vi "GetSetParameterValues.vi"(0 "VISA resource name":refnum<visa-resource-name>, 1 "get/set":T4, 2 "Control channel number (1-4)":T3=1 items=["Channel 1"=1, "Channel 2"=2, "Channel 3"=3, "Channel 4"=4], 3 "Parameter group number (1-4)":u8=1 min=1 max=4 step=1, 4 "Select Non-PTC(F) or PTC(T)":bool, 5 "error in":errorcluster, 6 "Non-PTC operation":T2 {"Cool IT" max=1000 step=1; "Cool PB" min=0 max=9999 step=1 format="%0.1f"; "Cool TL" min=-100 max=0 step=1 format="%0.1f"; "Heat TL" min=0 max=100 step=1 format="%0.1f"; "Heat IT" max=1000 step=1; "Heat PB" min=0 max=9999 step=1 format="%0.1f"}, 7 "PTC operation":T1 {"Cool IT" max=1000 step=1; "Cool Gain" min=0 max=9999 step=1 format="%0.1f"; "Cool Off" min=-100 max=0 step=1 format="%0.1f"; "Heat Off" min=0 max=100 step=1 format="%0.1f"; "Heat IT" max=1000 step=1; "Heat Gain" min=0 max=9999 step=1 format="%0.1f"}) -> (14 "VISA resource name out":refnum<visa-resource-name>, 15 "Parameter values response":string, 19 "error out":errorcluster)   [LabVIEW 2023, in "Thermotron 8800.lvlib"]
doc: "PARM\nCAUTION: This command is included for advanced users. Changing parameter group settings can adversely affect chamber control.\nCommand name: Send or load parameter values\nCommand type: Variable\nDescription: The query command causes the 8800 to send the values of the tuning parameters for the selected channel in the selected parameter group. The operation command sends new parameter values for a selected channel of a selected parameter group. The 8800 loads the parameter values into the parameter group registers in any mode. NOTE: When using the operation command, you must specify values for every field and not leave any field blank.\nQuery syntax: PARMc, g?\nWhere c = control channel number (1 through 4) and g = parameter group number (1 through 4).\nNon-PTC operation: PARMc, g, hpb, cpb, hit, cit, htl, ctl\nWhere:\nc Control channel number (1 through 4)\ng Parameter group number (1 through 4)\nhpb/cpb Heat and cool proportion bands (0.0 – 9999.0)\nhit/cit Heat and cool integral time (0 to 1000 seconds)\nhtl Heat throttle limit (0.0 to 100.0)\nctl Cool throttle limit (-100.0 to 0.0)\nPTC operation: PARMc, g, hgn, cgn, hit, cit, hof, cof\nWhere:\nc Control channel number (1 through 4)\ng Parameter group number (1 through 4)\nhgn/cgn Heat and cool gain settings for PTC operations (0.0 – 9999.0)\nhit/cit Heat and cool integral time (0 to 1000 seconds)\nhof Heat offset (0.0 to 100.0)\ncof Cool offset (-100.0 to 0.0)\nData type: Integer\nQuery example: PARM2,3?\n8800 response: 35.0,35.0,200,200,100.0,-100.0 (The channel 2 parameter group 3 settings are: heat and cool proportion bands 35.0, heat and cool integral times 200, heat throttle limit 100.0, and cool throttle limit -100.0.)\nOperation example: Non-PTC: To set the channel 1 parameter group 1 cool proportional band to 35.7 and keep the other channel 1 group 1 parameters at their factory values, send: PARM1,1,20,35.7,60,90,100.0,-100.0.\nPTC: With channel 4 in PTC mode, send the following command to set the channel 4 group 1 heat gain to 0.8, cool integral time to 128 seconds, and cool offset to 12.0, keeping the other channel 4 group 1 parameters at their factory values: PARM4,1,0.8,3.0,200,128,10.0,-12.0."
uses:
  Thermotron 8800.lvlib
  Private/get set.ctl
  Private/AnalogInputChannelNumber 1-4.ctl
panel:
  # "Gain settings for PTC operations (0.0-9999.0)"
  # "Integral time for PTC (0-1000 seconds)"
  # "Offset (0.0 - 100.0)"
  # "Proportional bands (0.0-9999.0)"
  # "Integral time (0 - 1000 seconds )"
  # "Throttle limit (0.0 - 100.0)"
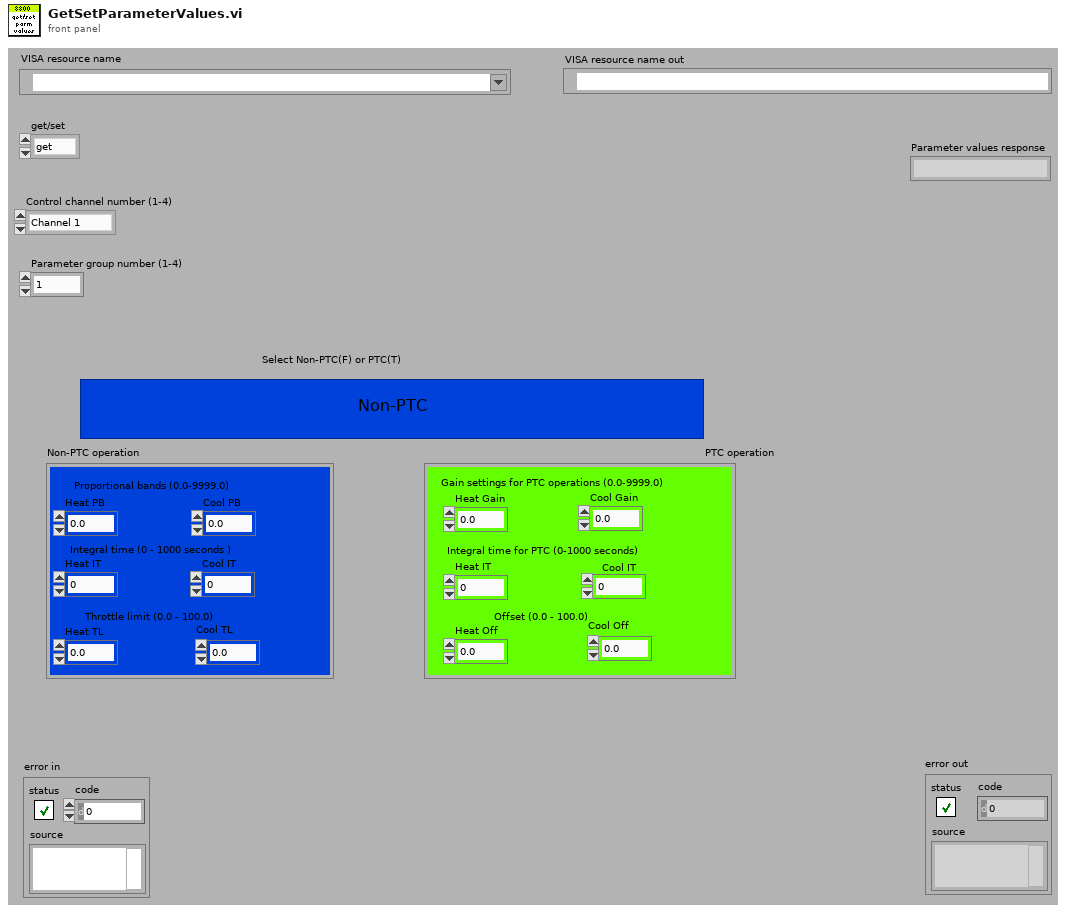
[diagram p1: front panel]
types:
  T1 = cluster{"Heat Gain":sgl, "Heat IT":u16, "Heat Off":sgl, "Cool Off":sgl, "Cool Gain":sgl, "Cool IT":u16}
  T2 = cluster{"Heat PB":sgl, "Heat IT":u16, "Heat TL":sgl, "Cool TL":sgl, "Cool PB":sgl, "Cool IT":u16}
  T3 = typedef "Thermotron 8800.lvlib/AnalogInputChannelNumber 1-4.ctl" = u16
  T4 = typedef "Thermotron 8800.lvlib/get set.ctl" = enum16{"get", "set"}
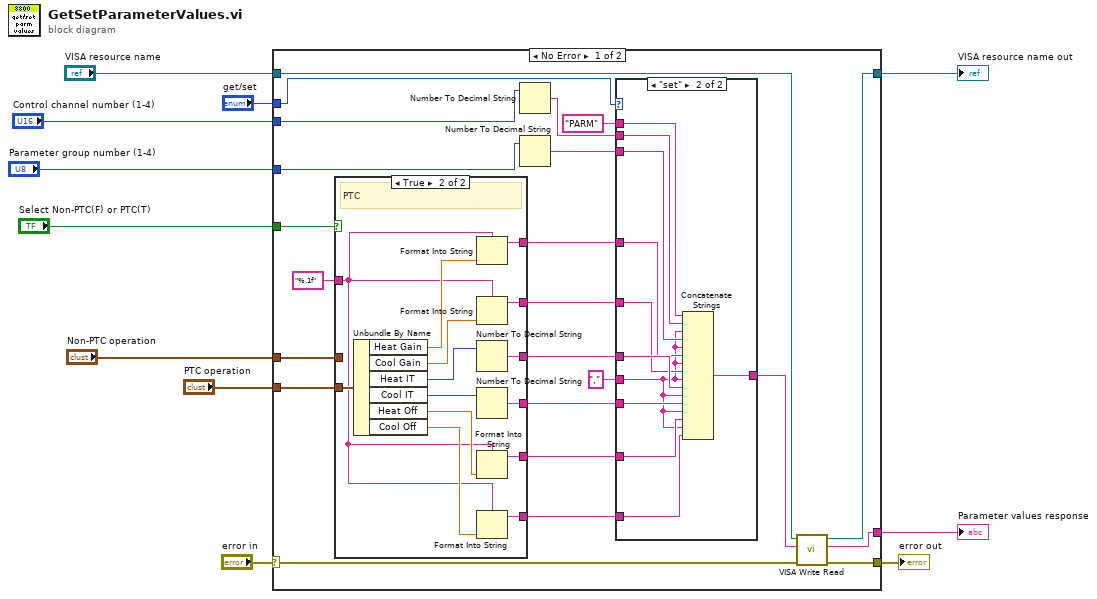
[diagram p0: block diagram]
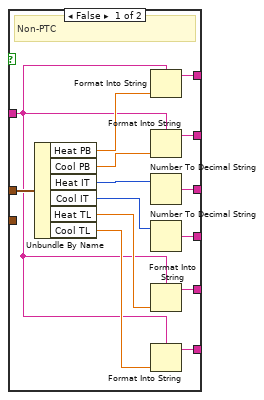
[diagram p2: hidden frame]
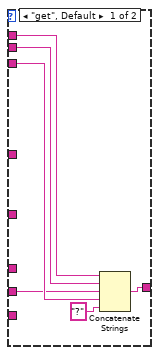
[diagram p3: hidden frame]
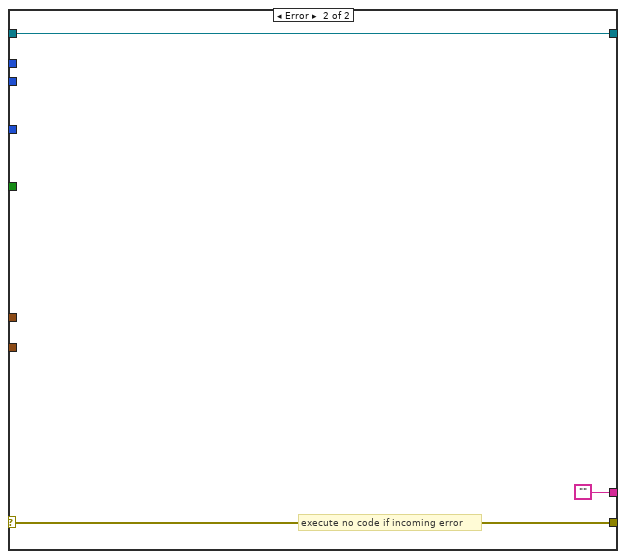
[diagram p4: hidden frame]
diagram:
  n1 = case shown="No Error" "error in" {
    selector: "error in" -> [w34 w81]
    tunnel: [w31 w82] -> w10
    tunnel: "VISA resource name" -> [w32 w82]
    tunnel: [w33 w81] -> w8
    tunnel: [w30 ""] -> w7
    tunnel: "get/set" -> [w29 _]
    tunnel: "Parameter group number (1-4)" -> [w25 _]
    tunnel: "PTC operation" -> [w20 _]
    tunnel: "Non-PTC operation" -> [w21 _]
    tunnel: "Control channel number (1-4)" -> [w26 _]
    tunnel: "Select Non-PTC(F) or PTC(T)" -> [w27 _]
    frame No Error {
      n2 = case shown="True" w27 {
        tunnel: w21 -> [w48 _]
        tunnel: w20 -> [_ w62]
        tunnel: [w46 w60] -> w19
        tunnel: [w44 w58] -> w18
        tunnel: [w42 w56] -> w17
        tunnel: [w40 w54] -> w16
        tunnel: [w38 w52] -> w15
        tunnel: [w36 w50] -> w14
        tunnel: "%.1f" ("format string") -> [w35 w49]
        frame False {
          # "Non-PTC"
          n3 = Unbundle By Name(w48) -> ("Heat PB"=w47:sgl, "Cool PB"=w45:sgl, "Heat IT"=w43:u16, "Cool IT"=w41:u16, "Heat TL"=w39:sgl, "Cool TL"=w37:sgl)
          n4 = Format Into String(format string=w35, w47) -> (resulting string=w46:string)  [unwired: 2 in, 1 out]
          n5 = Format Into String(format string=w35, w45) -> (resulting string=w44:string)  [unwired: 2 in, 1 out]
          n6 = Number To Decimal String(number=w43) -> (decimal integer string=w42:string)  [unwired: 1 in]
          n7 = Number To Decimal String(number=w41) -> (decimal integer string=w40:string)  [unwired: 1 in]
          n8 = Format Into String(format string=w35, w39) -> (resulting string=w38:string)  [unwired: 2 in, 1 out]
          n9 = Format Into String(format string=w35, w37) -> (resulting string=w36:string)  [unwired: 2 in, 1 out]
        }
        frame True {
          # "PTC"
          n10 = Unbundle By Name(w62) -> ("Heat Gain"=w61:sgl, "Cool Gain"=w59:sgl, "Heat IT"=w57:u16, "Cool IT"=w55:u16, "Heat Off"=w53:sgl, "Cool Off"=w51:sgl)
          n11 = Format Into String(format string=w49, w61) -> (resulting string=w60:string)  [unwired: 2 in, 1 out]
          n12 = Format Into String(format string=w49, w59) -> (resulting string=w58:string)  [unwired: 2 in, 1 out]
          n13 = Number To Decimal String(number=w57) -> (decimal integer string=w56:string)  [unwired: 1 in]
          n14 = Number To Decimal String(number=w55) -> (decimal integer string=w54:string)  [unwired: 1 in]
          n15 = Format Into String(format string=w49, w53) -> (resulting string=w52:string)  [unwired: 2 in, 1 out]
          n16 = Format Into String(format string=w49, w51) -> (resulting string=w50:string)  [unwired: 2 in, 1 out]
        }
      }
      n17 = Number To Decimal String(number=w26) -> (decimal integer string=w24:string)  [unwired: 1 in]
      n18 = Number To Decimal String(number=w25) -> (decimal integer string=w23:string)  [unwired: 1 in]
      n19 = case shown="\"set\"" w29 {
        tunnel: "PARM" ("8800 Command") -> [w68 w79]
        tunnel: [w67 w78] -> w12
        tunnel: w24 -> [w65 w77]
        tunnel: w23 -> [w64 w76]
        tunnel: "," ("8800 Command") -> [w63 w69]
        tunnel: w19 -> [_ w70]
        tunnel: w18 -> [_ w71]
        tunnel: w17 -> [_ w72]
        tunnel: w16 -> [_ w73]
        tunnel: w15 -> [_ w74]
        tunnel: w14 -> [_ w75]
        frame "get", Default {
          n20 = Concatenate Strings(w68, w65, w63, w64, "?" ("8800 Command")) -> (w67:string)
        }
        frame "set" {
          n21 = Concatenate Strings(w79, w77, w69, w76, w69, w70, w69, w71, w69, w72, w69, w73, w69, w74, w69, w75) -> (w78:string)
        }
      }
      n22 = call "VISA Write Read.vi"("error in (no error)"=w34, "8800 Command"=w12, "VISA Refnum in"=w32) -> ("error out"=w33:errorcluster, "read buffer"=w30:string, "VISA Refnum out"=w31:refnum<visa-resource-name>)  [unwired: 6 in]
    }
    frame Error {
      # "execute no code if incoming error"
    }
  }
  "VISA resource name out" <- w10
  "error out" <- w8
  "Parameter values response" <- w7
